vi "RMAD traffic control.vi"() -> ()   [LabVIEW 2017]
panel:
  out "mast mot trafikklys output array":i32[](array[numeric])
  out "abort":bool
  out "tcp sting":string
  out "Stredstørrelser terskelverdier":T1(array[cluster])
  out "mac adresses":T2
  out "init cluster":cluster{bool[], bool[]}
  out "num nodes":u32
  in  "Tab Control":enum32{"Status", "Siste Hendelser", "Config"}(tab)
  out "Status":bool[](array[boolean])
  out "Skred i skredløp":bool[][](array[boolean])
  out "Skred":bool[](array[boolean])
  out "Online":bool[](array[boolean])
  out "Aktiv":bool[](array[boolean])
  out "puls":bool
  out "trafikkvarsling enabled":bool
  out "SMS":bool[](array[boolean])
  out "sms enabled":bool
  out "Sensornavn":string[](array[string])
  out "Siste registrerte skred (sensor)":T3(array[cluster]) {"Intensitet terskel 1" format="%.1f"; "Intensitet terskel 2" format="%.1f"; "Intensitet terskel 3" format="%.1f"; "Intensitet terskel 4" format="%.1f"; "Intensitet terskel 5" format="%.1f"}
  in  "sms test":bool
  out "Debug Main":errorcluster
  out "up time (W:D:H)":dbl format="%<%W:%D:%H:%M:%S>t"
  out "gateway IP":T4={"serial_mux IP"="127.0.0.1", "serial_mux port"=9900}
  out "sec since last packet":dbl
  out "Debug overvåking":errorcluster
  out "TCP loop":i32
  out "ini file":path
  out "Trafikkontroll terskelverdier (sensor)":T5(array[cluster])
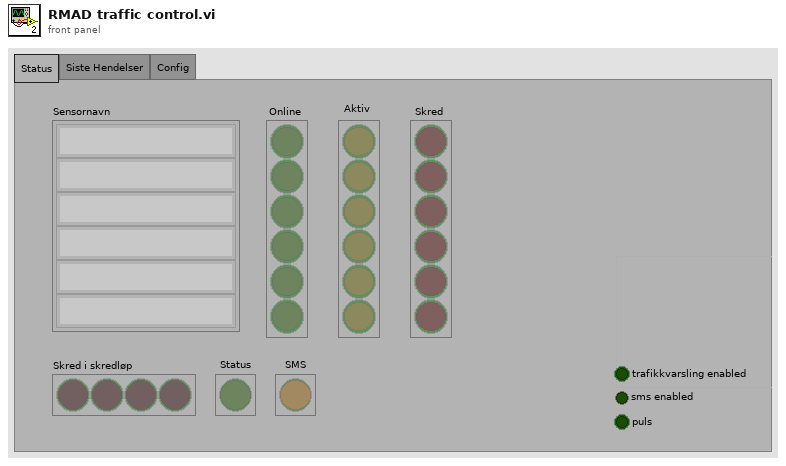
[diagram p1: front panel]
types:
  T1 = cluster{"teskelverdi":u32, "antall sensorer":u32, "varighet":u32}[][]
  T2 = cluster{"dust master mac":string, "xbee master mac":string, "master name":string, "dust mac":string[], "xbee mac":string[], "node names":string[]}
  T3 = cluster{"Tidspungt (mesh)":timestamp, "Skredstørrelse":u16, "Trafikklys":bool, "Antall pakker totalt":u16, "Varighet terskel 1":u16, "Intensitet terskel 1":dbl, "Varighet terskel 2":u16, "Intensitet terskel 2":dbl, "Varighet terskel 3":u16, "Intensitet terskel 3":dbl, "Varighet terskel 4":u16, "Intensitet terskel 4":dbl, "Varighet terskel 5":u16, "Intensitet terskel 5":dbl, "Mast Trigg":bool[], "Event ID":i32}[]
  T4 = cluster{"serial_mux IP":string, "serial_mux port":u16}
  T5 = cluster{"Intensitet":u32, "Antall geofoner":u32, "Varighet (s)":u32}[]
  T6 = cluster{"Device Health Report":cluster{"MAC adress":string, "charge (mC)":u32, "queueOcc":u8, "temperature (C)":i8, "batteryVoltage (mV)":u16, "numTxOk":u16, "numTxFail":u16, "numRxOK":u16, "numRxFail":u16, "numMACdropped":u8, "numTxBad":u8, "badLinkFrameID":u8, "badLinkSlot":u32, "badLinkOffset":u8}, "mote staus event":cluster{"data":string, u8}, "getMoteInfo":cluster{"MAC adress":string, "state":u8, "numNbrs":u8, "numGoodNbrs":u8, "requestedBw":u32, "totalNeededBw":u32, "assignedBw":u32, "packetsRecived":u32, "packetsLost":u32, "avgLatecy":u32}, "GetPathInfo":cluster{"Path ID":u8, "Src MAC":string, "Dest MAC":string, "direction":u8, "numLinks":u8, "quality":u8, "rssiScrDest":i8, "rssiDestScr":i8}, "Neighbors Health Report":cluster{"MAC adress":string, "neighbourHRdata":cluster{"neighbourID":u16, "neighborFlag":u8, "rssi":i8, "numTxPackets":u16, "numTxFailures":u16, "numRxPackets":u16}[]}, "Discovered Nighbors Health Report":cluster{"MAC adress":string, "numJoinParents":u8, cluster{"neighborID":u16, "rssi":i8, "numRx":u8}[]}, "Mote Config":cluster{"mac adress":string, "MoteID":u16, "isAP":bool, "mote state":u8, "reserved":u8, "isRouting":bool}}
  T7 = cluster{"MAc Adress":string, "UTC Time":timestamp, "srcPort":u16, "dstPort":u16, "data":string}
  T8 = cluster{"mac adress":string, "mote state":u8, "temperature (C)":i8, "battery (mV)":u16, "avg latecy":u32, "requested bw":u32, "good neighbour":u8, "num neighbour":u8, "num lost packets":u8, "last update (pc)":timestamp}[]
  T9 = cluster{"ID":u16, "Timestamp":timestamp, "Packets":u16, "SPS":dbl, "Samples":u16}[][]
  T10 = cluster{"Is logging":bool, "num avalanch":u16, "logging startet":timestamp}[]
  T11 = cluster{"Dust Timestamp":timestamp, "Limit reached flagg":bool[], "A1 std":sgl, "A2 std":sgl, "A3 std":sgl, "A4 std":sgl, "A1 rat":sgl, "A2 rat":sgl, "A3 rat":sgl, "A4 rat":sgl, "A1 max":u16, "A2 max":u16, "A3 max":u16, "A4 max":u16, "A1 min":u16, "A2 min":u16, "A3 min":u16, "A4 min":u16, "A1 maxS":u16, "A2 maxS":u16, "A3 maxS":u16, "A4 maxS":u16, "A1 minS":u16, "A2 minS":u16, "A3 minS":u16, "A4 minS":u16}[]
  T12 = cluster{"terskelverdi":u32, "antall sensorer":u32, "varighet":u32}[]
  T13 = cluster{"serial_mux IP":string, "rserial_mux port":u16}
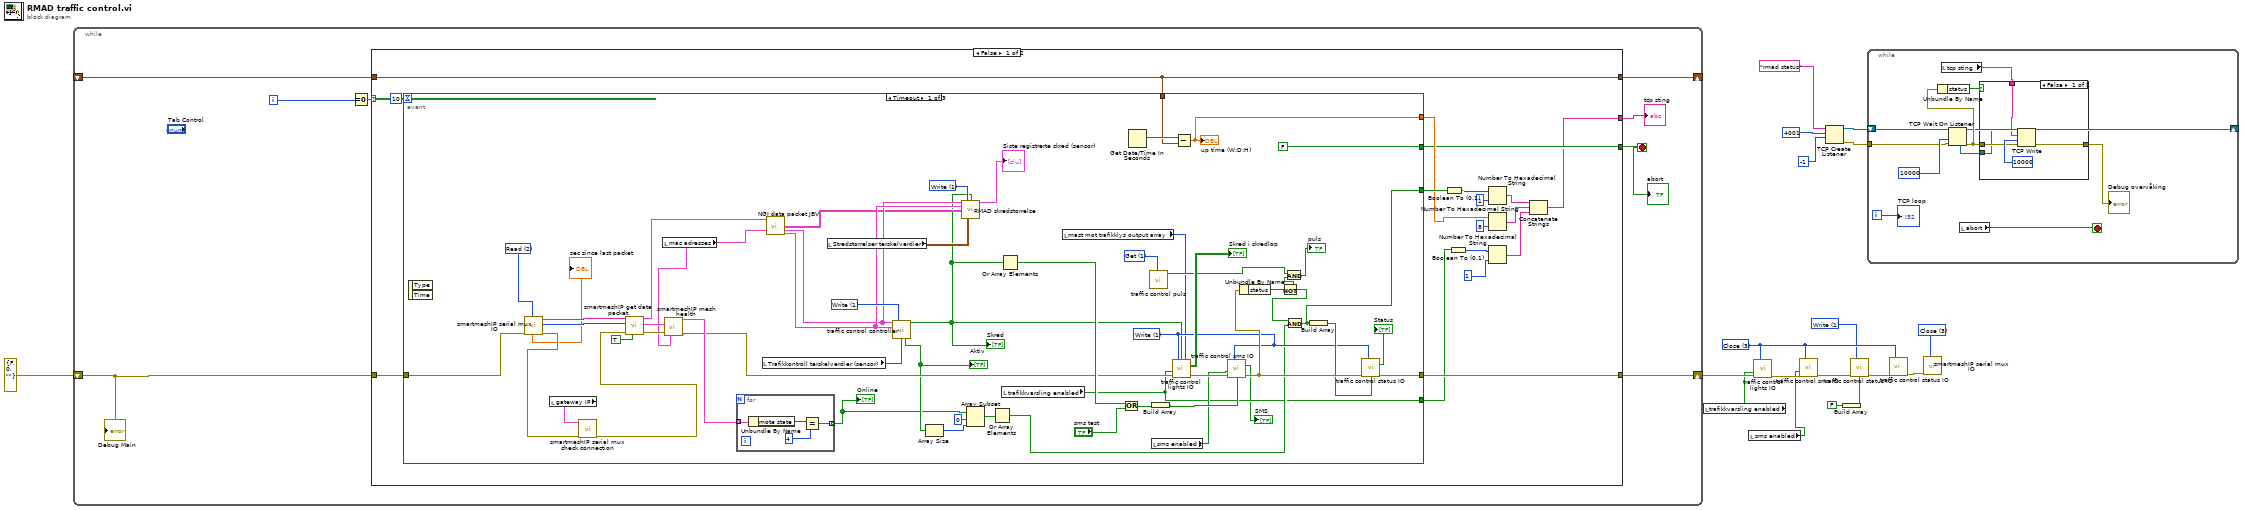
[diagram p0: block diagram]
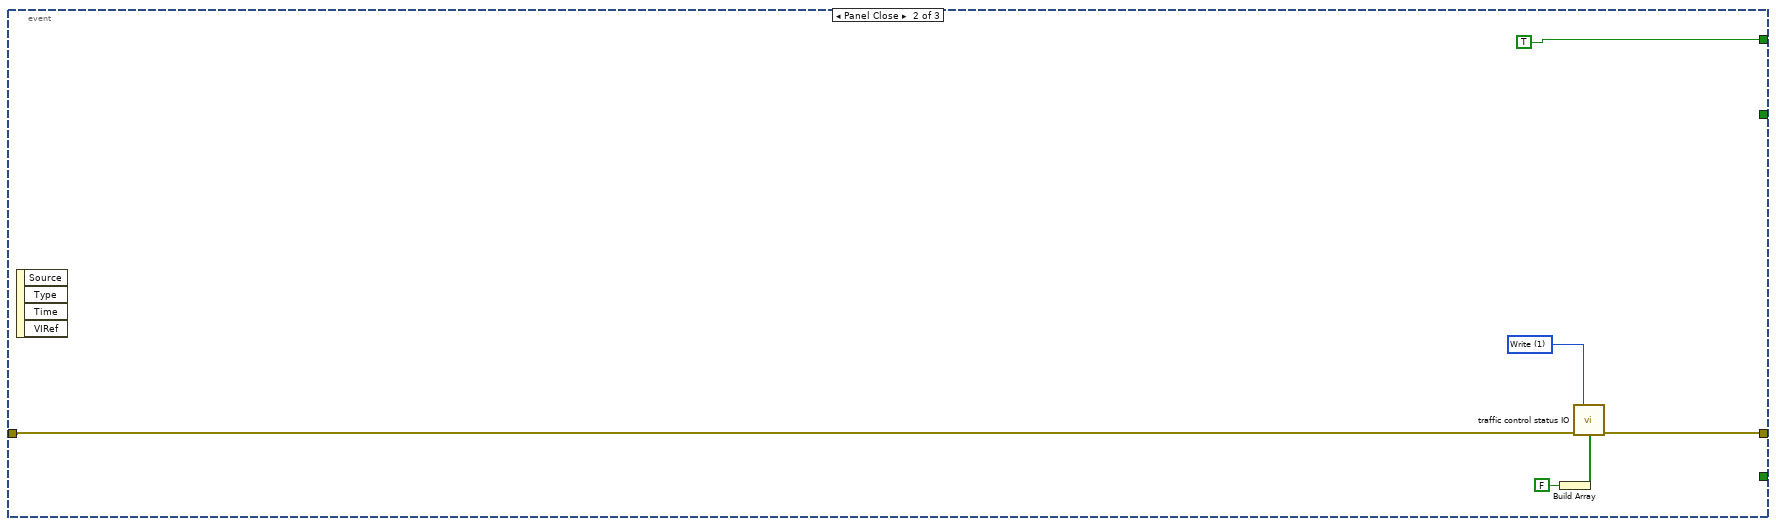
[diagram p3: hidden frame]
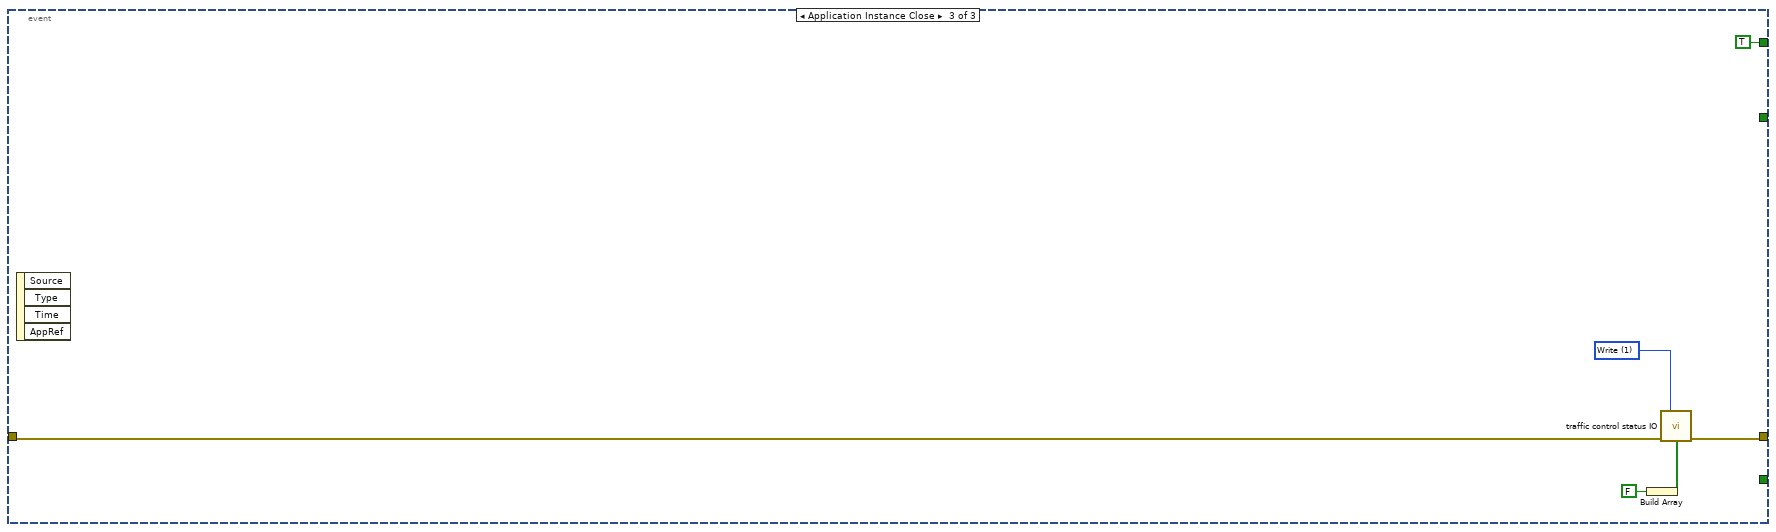
[diagram p4: hidden frame]
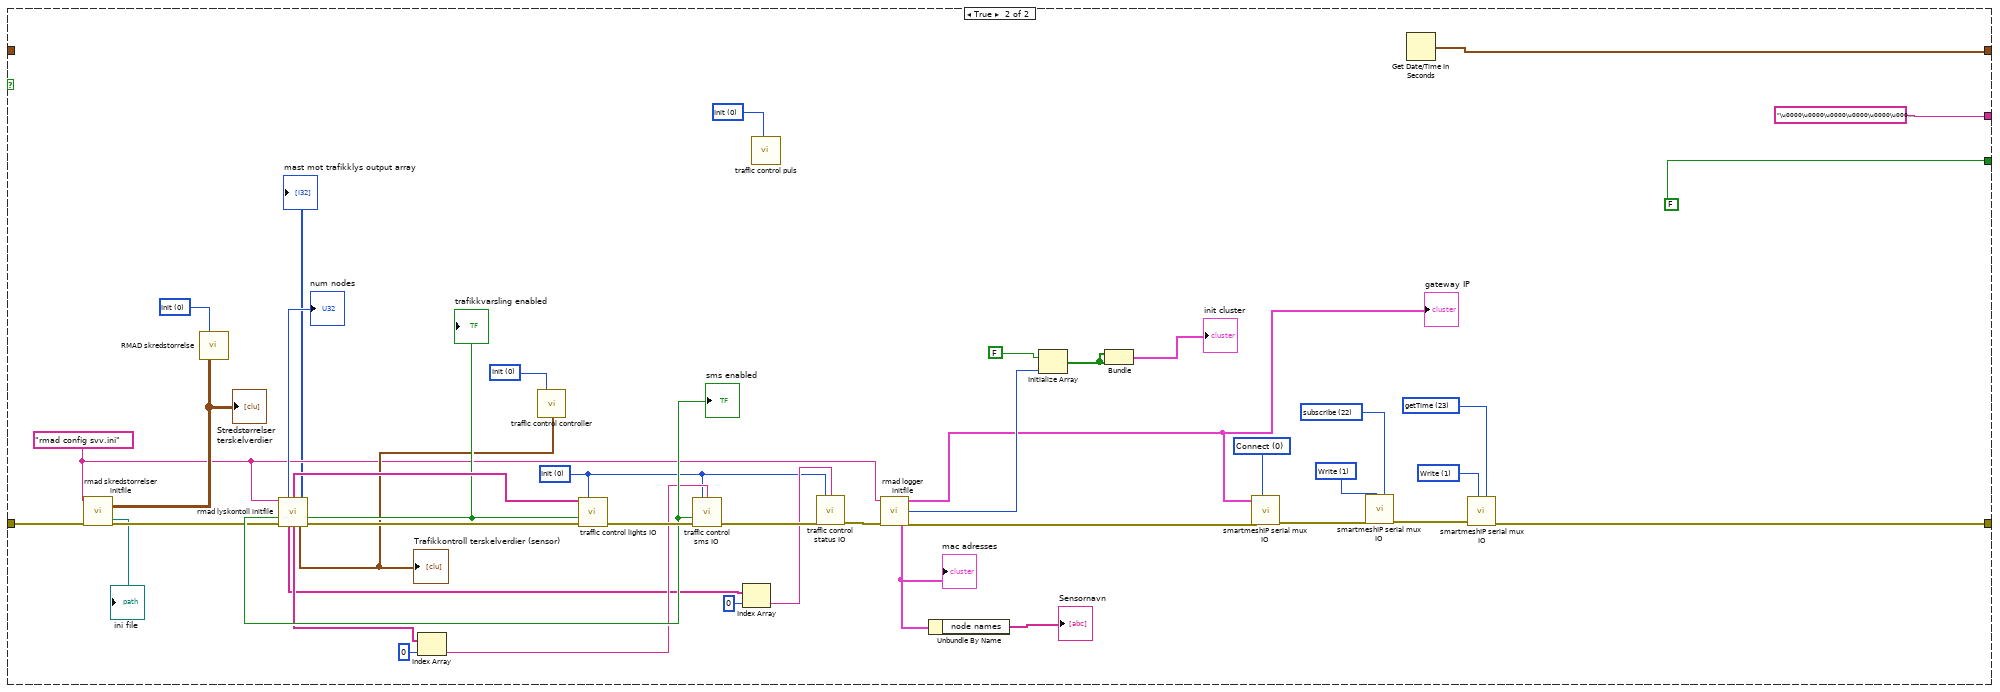
[diagram p5: hidden frame]
diagram:
  w8 = u16 1 items=["Init", "Write", "Read", "Close"] ("state")
  w11 = u16 3 items=["Init", "Write", "Read", "Close"] ("state")
  w18 = u16 3 items=["Connect", "Write", "Read", "Close"] ("State")
  n1 = while {
    shift-right: [w23] -> w16
    shift-left: errorcluster {"status"=FALSE, "code"=0, "source"=""} ("error out") -> [w22]
    shift-right: [w25] -> _
    shift-left: _ -> [w24]
    i -> [w21]
    stop <- w20 stop-if-true
    n2 = Equal To 0?(x=w21) -> (x = 0?=w26:bool)
    n3 = case shown="False" w26 {
      tunnel: [w35 w119] -> w23
      tunnel: w22 -> [w42 w125]
      tunnel: [w32 FALSE] -> w20
      tunnel: [w41 w145] -> w25
      tunnel: w24 -> [w41 _]
      tunnel: [w31 "\u0000\u0000\u0000\u0000\u0000\u0000\u0000\u0000\u0000\u0000"] -> w19
      frame False {
        n4 = event shown="[0] Timeout" {
          selector: _ -> [_ _ _]
          dyn-events: _ -> [_ _ _]
          timeout: 10 -> [_ _ _]
          tunnel: [w65 w104 w110] -> w35
          tunnel: w42 -> [w95 w103 w109]
          tunnel: [FALSE TRUE TRUE] -> w32
          tunnel: w41 -> [w92 _ _]
          tunnel: [w55 _ _] -> w40
          tunnel: [w54 _ _] -> w33
          tunnel: [w48 _ _] -> w30
          event Timeout {
            w70 = u16 1 items=["Init", "Write"] ("State")
            w86 = u16 1 items=["Init", "Get"] ("state")
            w96 = u16 2 items=["Connect", "Write", "Read", "Close"] ("State")
            w63 = u16 1 items=["Init", "Write", "Read", "Close"] ("state")
            w98 = u16 1 items=["Init", "Write", "Read", "Close"] ("State")
            n5 = event-data() -> ()  [unwired: 1 in, 2 out]
            n6 = call "smartmeshIP serial mux IO.vi"("State"=w96, "error in"=w95) -> ("error out"=w84:errorcluster, "rx_commandType"=w91:u8, "rx_data"=w90:string, "sec since last packet"=→"sec since last packet":dbl)  [unwired: 4 in, 2 out]
            n7 = local read "gateway IP"() -> (w85:T4)
            n8 = call "smartmeshIP serial mux check connection.vi"("error in"=w84, "serial mux adress"=w85) -> ("error out"=w83:errorcluster)  [unwired: 8 in, 1 out]
            n9 = call "smartmeshIP get data packet.vi"("use correction"=TRUE, "error in"=w83, "commandType"=w91, "data"=w90) -> ("error out"=w87:errorcluster, "mote and link status"=w88:T6, "Data Notifications"=w53:T7)  [unwired: 5 in]
            n10 = local read "mac adresses"() -> (w52:T2)
            n11 = call "smartmeshIP mesh health.vi"("mote and link status"=w88, "error in"=w87, "mac adresses"=w52) -> ("Mote Status"=w89:T8, "error out"=w67:errorcluster)  [unwired: 7 in, 4 out]
            n12 = for {
              tunnel: w89 -> [w102] mode=indexing
              tunnel: [w99] -> w61 mode=indexing
              n13 = Unbundle By Name(w102) -> ("mote state"=w101:u8)
              n14 = Equal?(x=w101, y=u8 4) -> (x = y?=w99:bool)
            }
            "Online" <- w61
            n15 = local read "Trafikkontroll terskelverdier (sensor)"() -> (w71:T5)
            n16 = call "NGI data packet JBV.vi"("Dust Data Notifications"=w53, "mac adresses"=w52) -> ("Recent events"=w49:T9, "Is Logging"=w50:T10, "Avalanch Packets"=w51:T11)  [unwired: 4 in, 7 out]
            n17 = local read "Stredstørrelser terskelverdier"() -> (w68:T1)
            n18 = call "traffic control controller.vi"("Is Logging"=w50, "State"=w98, "Avalanch Packets"=w51, "Trafikkontroll terskelverdier"=w71) -> ("Rød mast"=w47:bool[], "Is Logging"=w62:bool[])  [unwired: 9 in, 1 out]
            "Skred" <- w47
            "Aktiv" <- w62
            n19 = Array Size(array=w62) -> (size(s)=w60:i32)
            n20 = call "RMAD skredstorrelse.vi"("Is Logging"=w50, "State"=w70, "Rød signal kriterie"=w47, "Avalanch Packets"=w51, "Recent events"=w49, "Stredstørrelser terskelverdier"=w68) -> ("Skredhendelser"=→"Siste registrerte skred (sensor)":T3)  [unwired: 5 in, 4 out]
            n21 = Array Subset(array=w61, index=0, length=w60) -> (w58:bool[])
            n22 = Or Array Elements(Boolean array=w58) -> (logical OR=w56:bool)
            n23 = Or Array Elements(Boolean array=w47) -> (logical OR=w72:bool)
            n24 = local read "trafikkvarsling enabled"() -> (w48:bool)
            n25 = local read "mast mot trafikklys output array"() -> (w46:i32[])
            n26 = Or(x=w72, y="sms test") -> (x .or. y?=w80:bool)
            n27 = Get Date/Time In Seconds() -> (seconds since 1Jan1904=w93:timestamp)
            n28 = call "traffic control puls.vi"("state"=w86) -> ("puls"=w75:bool)  [unwired: 10 in]
            n29 = Build Array(w80) -> (w78:bool[])
            n30 = local read "sms enabled"() -> (w77:bool)
            n31 = call "traffic control lights IO.vi"("state"=w63, "skred detektert av mast"=w47, "Mast vs skredløp output"=w46, "enable signallys"=w48, "error in"=w67) -> ("røde lys indikator"=→"Skred i skredløp":bool[][], "error out"=w79:errorcluster)  [unwired: 9 in]
            n32 = Subtract(x=w93, y=w92) -> (x-y=w54:dbl)
            "up time (W:D:H)" <- w54
            n33 = call "traffic control sms IO.vi"("state"=w63, "enable sms"=w77, "error in"=w79, "sms"=w78) -> ("sms indikator"=→"SMS":bool[], "error out"=w66:errorcluster)  [unwired: 10 in]
            n34 = Unbundle By Name(w66) -> ("status"=w76:bool)
            n35 = Not(x=w76) -> (.not. x?=w57:bool)
            n36 = And(x=w75, y=w57) -> (x .and. y?=→"puls":bool)
            n37 = And(x=w57, y=w56) -> (x .and. y?=w55:bool)
            n38 = Build Array(w55) -> (w64:bool[])
            n39 = call "traffic control status IO.vi"("state"=w63, "error in"=w66, "status"=w64) -> ("status indikator"=→"Status":bool[], "error out"=w65:errorcluster)  [unwired: 11 in]
          }
          event Panel Close {
            w107 = u16 1 items=["Init", "Write", "Read", "Close"] ("state")
            n40 = event-data() -> ()  [unwired: 1 in, 4 out]
            n41 = Build Array(FALSE) -> (w105:bool[])
            n42 = call "traffic control status IO.vi"("state"=w107, "error in"=w103, "status"=w105) -> ("error out"=w104:errorcluster)  [unwired: 11 in, 1 out]
          }
          event Application Instance Close {
            w113 = u16 1 items=["Init", "Write", "Read", "Close"] ("state")
            n43 = event-data() -> ()  [unwired: 1 in, 4 out]
            n44 = Build Array(FALSE) -> (w111:bool[])
            n45 = call "traffic control status IO.vi"("state"=w113, "error in"=w109, "status"=w111) -> ("error out"=w110:errorcluster)  [unwired: 11 in, 1 out]
          }
        }
        n46 = Boolean To (0,1)(Boolean=w40) -> (0, 1=w39:i16)
        n47 = Boolean To (0,1)(Boolean=w30) -> (0, 1=w29:i16)
        n48 = Number To Hexadecimal String(1:i16 1 ("width (-)"), 2:w39) -> (0:w37:string)
        n49 = Number To Hexadecimal String(1:i16 8 ("width (-)"), 2:w33) -> (0:w36:string)
        n50 = Number To Hexadecimal String(1:i16 1 ("width (-)"), 2:w29) -> (0:w27:string)
        n51 = Concatenate Strings(w37, w36, w27) -> (w31:string)
      }
      frame True {
        w116 = "rmad config svv.ini" ("initfile")
        w126 = u16 0 items=["Init", "Write"] ("State")
        w137 = u8 23 items=["subscribe"=22, "startNetwork"=45, "setUser"=58, "setTime"=54, "setNetworkConfig"=26, "setLicense"=56, "setIPConfig"=68, "setDownstreamFrameMode"=51, "setCommonJoinKey"=66, "setAdvertising"=50, "setACLEntry"=39, "sendIP"=59, "sendData"=44, "restorFactoryDefaults"=61, "reset"=21, "radiotestTx"=35, "radiotestRx"=37, "pingMote"=42, "getTime"=23, "getSystemInfo"=46, "radiotestStatistics"=38, "getPathInfo"=48, "getNextPath"=49, "getNextACLEntry"=40, "getNetworkInfo"=64, "getNetworkConfig"=63, "getMoteLinks"=70, "getMoteInfo"=62, "getMoteConfigByld"=65, "getMoteConfig"=47, "getManagerStatistics"=53, "getLog"=43, "getLicense"=55, "getIPConfig"=67, "exchangeNetworkID"=34, "exchangeMoteJoinKey"=33, "deleteMote"=69, "deleteACLEntry"=41, "clearStatistics"=31] ("commandType_write")
        w138 = u16 1 items=["Connect", "Write", "Read", "Close"] ("State")
        w144 = u16 0 items=["Init", "Get"] ("state")
        w150 = u8 22 items=["subscribe"=22, "startNetwork"=45, "setUser"=58, "setTime"=54, "setNetworkConfig"=26, "setLicense"=56, "setIPConfig"=68, "setDownstreamFrameMode"=51, "setCommonJoinKey"=66, "setAdvertising"=50, "setACLEntry"=39, "sendIP"=59, "sendData"=44, "restorFactoryDefaults"=61, "reset"=21, "radiotestTx"=35, "radiotestRx"=37, "pingMote"=42, "getTime"=23, "getSystemInfo"=46, "radiotestStatistics"=38, "getPathInfo"=48, "getNextPath"=49, "getNextACLEntry"=40, "getNetworkInfo"=64, "getNetworkConfig"=63, "getMoteLinks"=70, "getMoteInfo"=62, "getMoteConfigByld"=65, "getMoteConfig"=47, "getManagerStatistics"=53, "getLog"=43, "getLicense"=55, "getIPConfig"=67, "exchangeNetworkID"=34, "exchangeMoteJoinKey"=33, "deleteMote"=69, "deleteACLEntry"=41, "clearStatistics"=31] ("commandType_write")
        w149 = u16 1 items=["Connect", "Write", "Read", "Close"] ("State")
        w147 = u16 0 items=["Connect", "Write", "Read", "Close"] ("State")
        w127 = u16 0 items=["Init", "Write", "Read", "Close"] ("state")
        w158 = u16 0 items=["Init", "Write", "Read", "Close"] ("State")
        n52 = call "rmad skredstorrelser initfile.vi"("initfile"=w116, "error in (no error)"=w125) -> ("Stredstørrelser terskelverdier"=w123:T1, "ini file"=→"ini file":path, "error out"=w124:errorcluster)  [unwired: 9 in, 2 out]
        "Stredstørrelser terskelverdier" <- w123
        n53 = call "RMAD skredstorrelse.vi"("State"=w126, "Stredstørrelser terskelverdier"=w123) -> ()  [unwired: 9 in, 5 out]
        n54 = call "rmad lyskontoll initfile.vi"("init file"=w116, "error in (no error)"=w124) -> ("num geophone nodes"=→"num nodes":u32, "aktive skredløp"=w156:string[], "mast mot trafikklys output array"=→"mast mot trafikklys output array":i32[], "sms enabled"=w139:bool, "lights enables"=w155:bool, "status"=w129:string[], "sms"=w133:string[], "Trafikkontroll terskelverdier"=w120:T12, "error out"=w157:errorcluster)  [unwired: 5 in]
        "trafikkvarsling enabled" <- w155
        "sms enabled" <- w139
        "Trafikkontroll terskelverdier (sensor)" <- w120
        n55 = Index Array(array=w133, index=0) -> (element=w134:string)
        n56 = call "traffic control controller.vi"("State"=w158, "Trafikkontroll terskelverdier"=w120) -> ()  [unwired: 11 in, 3 out]
        n57 = call "traffic control lights IO.vi"("red channels"=w156, "state"=w127, "enable signallys"=w155, "error in"=w157) -> ("error out"=w140:errorcluster)  [unwired: 10 in, 1 out]
        n58 = call "traffic control sms IO.vi"("state"=w127, "eventch"=w134, "enable sms"=w139, "error in"=w140) -> ("error out"=w132:errorcluster)  [unwired: 10 in, 1 out]
        n59 = Index Array(array=w129, index=0) -> (element=w128:string)
        n60 = call "traffic control puls.vi"("state"=w144) -> ()  [unwired: 10 in, 1 out]
        n61 = call "traffic control status IO.vi"("state"=w127, "eventch"=w128, "error in"=w132) -> ("error out"=w131:errorcluster)  [unwired: 11 in, 1 out]
        n62 = call "rmad logger initfile.vi"("initfile"=w116, "error in (no error)"=w131) -> ("serial mux"=w142:T13, "num nodes"=w151:u32, "mac adresses"=w122:T2, "error out"=w141:errorcluster)  [unwired: 1 in, 9 out]
        "mac adresses" <- w122
        "gateway IP" <- w142
        n63 = Unbundle By Name(w122) -> ("node names"=→"Sensornavn":string[])
        n64 = Initialize Array(FALSE, w151) -> (w153:bool[])
        n65 = Bundle(w153, w153) -> (→"init cluster":cluster{bool[], bool[]})  [unwired: 1 in]
        n66 = call "smartmeshIP serial mux IO.vi"("State"=w147, "error in"=w141, "serial mux adress"=w142) -> ("error out"=w148:errorcluster)  [unwired: 3 in, 5 out]
        n67 = call "smartmeshIP serial mux IO.vi"("tx_commandType"=w150, "State"=w149, "error in"=w148) -> ("error out"=w136:errorcluster)  [unwired: 3 in, 5 out]
        n68 = Get Date/Time In Seconds() -> (seconds since 1Jan1904=w145:timestamp)
        n69 = call "smartmeshIP serial mux IO.vi"("tx_commandType"=w137, "State"=w138, "error in"=w136) -> ("error out"=w119:errorcluster)  [unwired: 3 in, 5 out]
      }
    }
    "tcp sting" <- w19
    "abort" <- w20
    "Debug Main" <- w22
  }
  n70 = local read "trafikkvarsling enabled"() -> (w15:bool)
  n71 = local read "sms enabled"() -> (w13:bool)
  n72 = call "traffic control lights IO.vi"("state"=w11, "enable signallys"=w15, "error in"=w16) -> ("error out"=w14:errorcluster)  [unwired: 11 in, 1 out]
  n73 = call "traffic control sms IO.vi"("state"=w11, "enable sms"=w13, "error in"=w14) -> ("error out"=w10:errorcluster)  [unwired: 11 in, 1 out]
  n74 = TCP Create Listener(9:-1 ("timeout ms (25000)"), 10:u16 4001 ("port"), 11:"rmad status" ("service name")) -> (0:w1:errorcluster, 3:w2:refnum<k5>)  [unwired: 2 in, 1 out]
  n75 = Build Array(FALSE) -> (w6:bool[])
  n76 = call "traffic control status IO.vi"("state"=w8, "error in"=w10, "status"=w6) -> ("error out"=w9:errorcluster)  [unwired: 11 in, 1 out]
  n77 = while {
    shift-right: [w163] -> _
    shift-left: w2 -> [w162]
    tunnel: w1 -> [w161]
    i -> [w164]
    stop <- w159 stop-if-true
    n78 = local read "tcp sting"() -> (w160:string)
    n79 = TCP Wait On Listener(8:w161, 9:10000 ("timeout ms (wait forever: -1)"), 11:w162) -> (0:w168:errorcluster, 3:w163:refnum<k5>, 4:w167:refnum<k5>)  [unwired: 1 in, 2 out]
    n80 = Unbundle By Name(w168) -> ("status"=w169:bool)
    n81 = local read "abort"() -> (w159:bool)
    n82 = case shown="False" w169 {
      tunnel: w160 -> [w173 _]
      tunnel: w168 -> [w172 w175]
      tunnel: w167 -> [w171 _]
      tunnel: [w170 w175] -> w165
      frame False {
        n83 = TCP Write(connection ID=w171, data in=w173, error in (no error)=w172, 9:10000 ("timeout ms (25000)")) -> (error out=w170:errorcluster)  [unwired: 2 out]
      }
      frame True {
      }
    }
    "Debug overvåking" <- w165
    "TCP loop" <- w164
  }
  n84 = call "traffic control status IO.vi"("state"=w11, "error in"=w9) -> ("error out"=w12:errorcluster)  [unwired: 12 in, 1 out]
  n85 = call "smartmeshIP serial mux IO.vi"("State"=w18, "error in"=w12) -> ()  [unwired: 4 in, 6 out]
